vi "Configure Acquisition.vi"(8 "error in (no error)":errorcluster, 11 "Thermometer DAQmx Base CFG in":refnum<class "Thermometer DAQmx Base CFG.lvclass">) -> (0 "error out":errorcluster, 3 "Thermometer DAQmx Base CFG out":refnum<class "Thermometer DAQmx Base CFG.lvclass">)   [LabVIEW 2023, in "Thermometer DAQmx Base CFG.lvclass"]
uses:
  Thermometer DAQmx Base CFG.lvclass
  Configuration/Configuration JSON/Configuration JSON Base/CFG JSON.lvclass/CFG JSON.ctl
  DAQmx/DAQmx Base CFG/DAQmx Base CFG.lvclass/DAQmx Base CFG.ctl
  dfb2f314-1d2b-4c7a-8d12-2ab81d0c55d9.vi
  <vilib>/JDP Science/JSONtext/Find Item.vi
  <vilib>/JDP Science/JSONtext/Next JSON Value.vi
  <vilib>/JDP Science/JSONtext/String Subset.vi
  <vilib>/JDP Science/JSONtext/Parsing/Advance past next JSON Value (inlined COPY).vi
  <vilib>/JDP Science/JSONtext/Parsing/Advance past whitespace.vi
  <vilib>/JDP Science/JSONtext/Parsing/Advance past String.vi
  <vilib>/JDP Science/JSONtext/Parsing/Advance past Number.vi
  <vilib>/JDP Science/JSONtext/Parsing/Advance past Line Ending.vi
  <vilib>/JDP Science/JSONtext/Parsing/Parse Full Path or Item Name.vi
  <vilib>/JDP Science/JSONtext/Parsing/Advance past Array.vi
  <vilib>/JDP Science/JSONtext/Parsing/Advance past Object.vi
  <vilib>/JDP Science/JSONtext/support/Error Cluster From Code.vi
  <vilib>/JDP Science/JSONtext/Offset/Find Item Locations by Path.vi
  <vilib>/JDP Science/JSONtext/JSON text to Variant.vi
  <vilib>/Utility/error.llb/Error Cluster From Error Code.vi
  <vilib>/JDP Science/JSONtext/LVClass Serializer/JSONtext LVClass Serializer.lvclass
  <vilib>/ErrorRing/Error Ring.xnode
  Thermometer DAQmx Base CFG.lvclass/Thermometer DAQmx Base CFG.ctl
  Configuration/Configuration JSON/Configuration JSON Base/CFG JSON.lvclass
  <resource>/objmgr/daqmx.rc
  DAQmx/DAQmx Base CFG/DAQmx Base CFG.lvclass
panel:
  out "OverWrite":i32(ring)=10159 items=["Overwrite Unread Samples"=10252, "Do Not Overwrite Unread Samples"=10159]
  out "RelativeTo":i32(ring)=10425 items=["First Sample"=10424, "Current Read Position"=10425, "Reference Trigger"=10426, "First Pretrigger Sample"=10427, "Most Recent Sample"=10428]
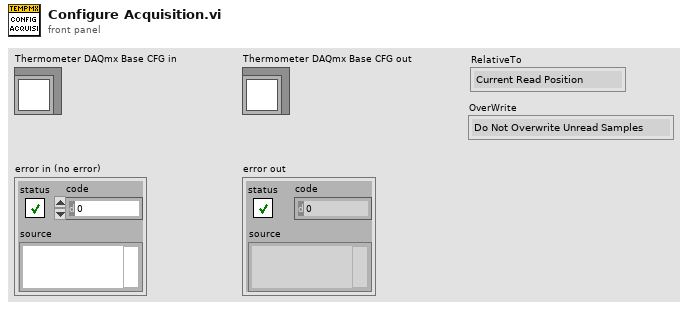
[diagram p1: front panel]
types:
  T1 = cluster{"Relative To":string, "Overwrite":string}
  T2 = typedef "LVStringsAndValuesArrayTypeDef_I32.ctl" = cluster{"String":string, "Value":i32}[]
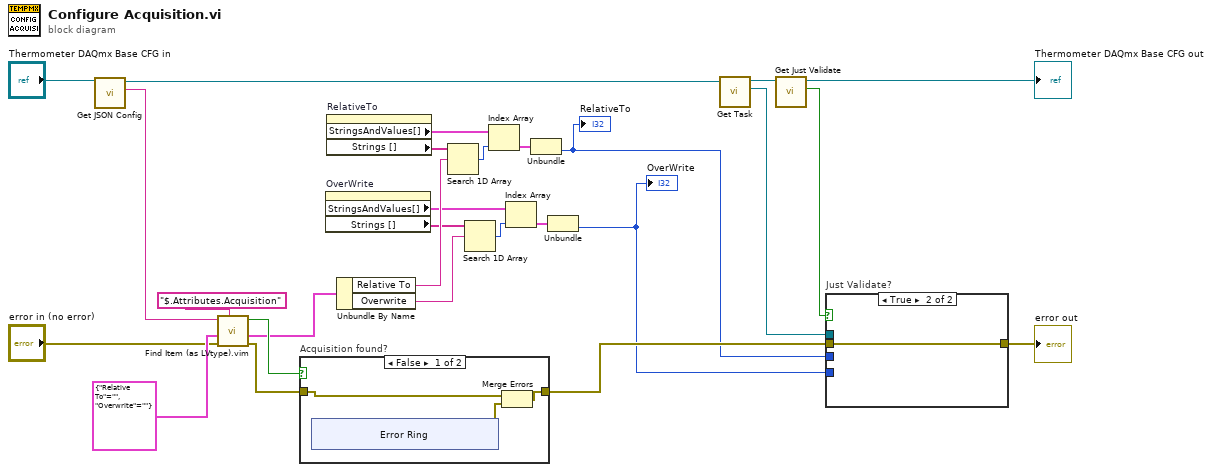
[diagram p0: block diagram]
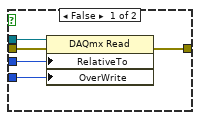
[diagram p3: hidden frame]
diagram:
  n1 = call "Get JSON Config.vi"("CFG Base in"="Thermometer DAQmx Base CFG in") -> ("<JSON>Config>"=w26:string, "CFG Base out"=w1:refnum<class "Thermometer DAQmx Base CFG.lvclass">)  [unwired: 9 in]
  n2 = call "Find Item (as LVtype).vim"("$Path or Item Name"="$.Attributes.Acquisition", "error in (no error)"="error in (no error)", "Data Type and Default Value"=T1 {"Relative To"="", "Overwrite"=""}, "JSON"=w26) -> ("error out"=w23:errorcluster, "Data"=w16:T1, "Found"=w24:bool)  [unwired: 4 in, 1 out]
  n3 = case "Acquisition found?" shown="False" w24 {
    tunnel: w23 -> [w30 w36]
    tunnel: [w28 w36] -> w22
    frame False {
      n4 = xnode "Error Ring"() -> ("error out"=w29:errorcluster)
      n5 = Merge Errors(w30, w29) -> (w28:errorcluster)
    }
    frame True {
    }
  }
  n6 = property on="OverWrite" class="Ring (strict)"() -> ("StringsAndValues[]"=w11:T2, "Strings []"=w10:string[])  [unwired: 2 in, 2 out]
  n7 = property on="RelativeTo" class="Ring (strict)"() -> ("StringsAndValues[]"=w19:T2, "Strings []"=w18:string[])  [unwired: 2 in, 2 out]
  n8 = Unbundle By Name(w16) -> ("Relative To"=w15:string, "Overwrite"=w9:string)
  n9 = Search 1D Array(1D array=w18, element=w15) -> (index of element=w20:i32)  [unwired: 1 in]
  n10 = Search 1D Array(1D array=w10, element=w9) -> (index of element=w12:i32)  [unwired: 1 in]
  n11 = Index Array(array=w19, index=w20) -> (element=w21:cluster{"String":string, "Value":i32})
  n12 = Index Array(array=w11, index=w12) -> (element=w13:cluster{"String":string, "Value":i32})
  n13 = Unbundle(w21) -> ("Value"=w14:i32)  [unwired: 1 out]
  "RelativeTo" <- w14
  n14 = Unbundle(w13) -> ("Value"=w8:i32)  [unwired: 1 out]
  "OverWrite" <- w8
  n15 = call "Get Task.vi"("DAQmx Base CFG in"=w1) -> ("Task"=w4:refnum<k21>, "DAQmx Base CFG out"=w5:refnum<class "Thermometer DAQmx Base CFG.lvclass">)  [unwired: 9 in]
  n16 = call "Get Just Validate.vi"("CFG JSON Base in"=w5) -> ("Just Validate"=w6:bool, "CFG JSON Base out"=→"Thermometer DAQmx Base CFG out":refnum<class "Thermometer DAQmx Base CFG.lvclass">)  [unwired: 9 in]
  n17 = case "Just Validate?" shown="True" w6 {
    tunnel: [w41 w42] -> w25
    tunnel: w4 -> [w40 _]
    tunnel: w22 -> [w39 w42]
    tunnel: w14 -> [w38 _]
    tunnel: w8 -> [w37 _]
    frame False {
      n18 = property class="DAQmx Read"(reference=w40, error in=w39, "RelativeTo"=w38, "OverWrite"=w37) -> (error out=w41:errorcluster)  [unwired: 1 out]
    }
    frame True {
    }
  }
  "error out" <- w25
